vi "UART Get Bytes Available.vi"(8 "Error In":errorcluster, 10 "UART Channel (0)":u8, 11 "LINX Resource":T1) -> (0 "Error Out":errorcluster, 1 "Bytes Available":u8, 3 "LINX Resource":T1)   [LabVIEW 2020, in "LMH-LINX.lvlib"]
doc: "Get the number of bytes available in the LINX device's UART receive buffer specified by UART Channel."
uses:
  LMH-LINX.lvlib
  Private/Type Defs/LINX Ref.ctl
  Private/Type Defs/Platform.ctl
  Private/Type Defs/Interface.ctl
  Private/Device/Type Defs/LINX Device Config.ctl
  Private/Device/Type Defs/TCP Config.ctl
  Private/Device/Type Defs/Channels.ctl
  Private/Type Defs/Peripheral.ctl
  Private/Utilties/Generate Error.vi
  Private/Device/Device.lvlib
  Private/Local IO/Local IO.lvlib
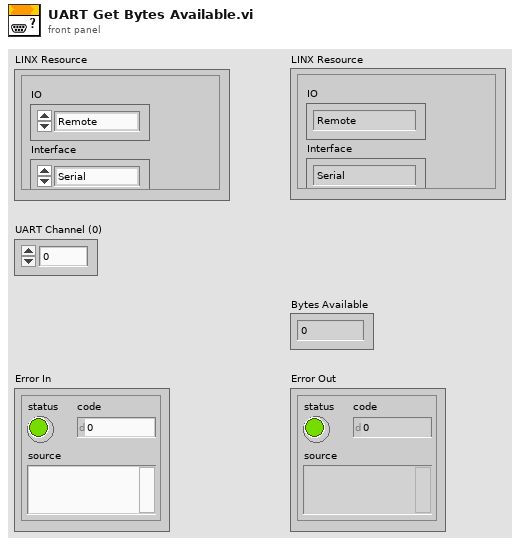
[diagram p1: front panel]
types:
  T1 = typedef "LMH-LINX.lvlib/LINX Ref.ctl" = cluster{"IO":T2, "Interface":T3, "LINX Device Config":T4}
  T2 = typedef "LMH-LINX.lvlib/Platform.ctl" = enum16{"Remote", "Local"}
  T3 = typedef "LMH-LINX.lvlib/Interface.ctl" = enum16{"Serial", "TCP"}
  T4 = typedef "Device.lvlib/LINX Device Config.ctl" = cluster{"Interface":T3, "COM Port":refnum<visa-resource-name>, "TCP Configuration":T5, "Device Family":u8, "Device ID":u8, "Device Name":string, "TCP Ref":refnum<k5>, "Channels":T6}
  T5 = typedef "Device.lvlib/TCP Config.ctl" = cluster{"IP Address":string, "Port":u16}
  T6 = typedef "LMH-LINX.lvlib/Channels.ctl" = cluster{"DI":u8[], "DO":u8[], "AI":u8[], "AO":u8[], "PWM":u8[], "QE":u8[], "UART":u8[], "I2C 2":u8[], "SPI":u8[], "CAN":u8[], "Servo":u8[], "AI Ref (V)":dbl, "AI Resolution (Bits)":u8, "AO Ref (V)":dbl, "AO Resolution (Bits)":u8}
  T7 = typedef "LMH-LINX.lvlib/Peripheral.ctl" = enum8{"DI", "DO", "AI", "AO", "PWM", "QE", "UART", "I2C", "SPI", "CAN", "Servo"}
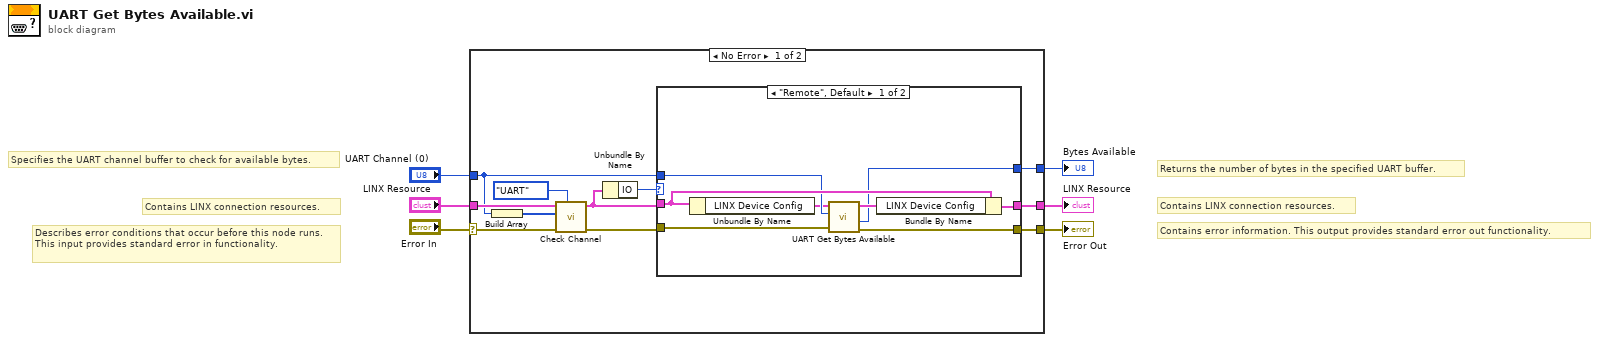
[diagram p0: block diagram]
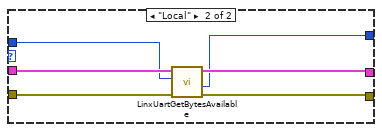
[diagram p2: hidden frame]
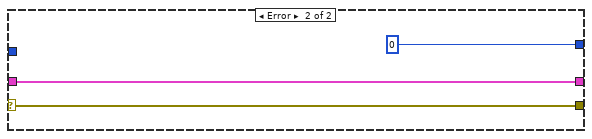
[diagram p3: hidden frame]
diagram:
  # "Returns the number of bytes in the specified UART buffer."
  # "Specifies the UART channel buffer to check for available bytes."
  # "Contains LINX connection resources."
  # "Contains error information. This output provides standard error out functionality."
  # "Contains LINX connection resources."
  # "Describes error conditions that occur before this node runs. This input provides standard error in functionality."
  n1 = case shown="No Error" "Error In" {
    selector: "Error In" -> [w7 w34]
    tunnel: [w16 w34] -> w6
    tunnel: [w15 w33] -> w5
    tunnel: "LINX Resource" -> [w14 w33]
    tunnel: "UART Channel (0)" -> [w10 _]
    tunnel: [w8 u8 0 ("Bytes at Port")] -> w2
    frame No Error {
      n2 = Build Array(w10) -> (w11:u8[])
      n3 = call "Check Channel.vi"("Peripheral"=Peripheral."UART", "Error In"=w7, "Channels"=w11, "LINX Resource"=w14) -> ("Error Out"=w12:errorcluster, "LINX Resource"=w13:T1)  [unwired: 5 in, 1 out]
      n4 = Unbundle By Name(w13) -> ("IO"=w17:T2)
      n5 = case shown="\"Remote\", Default" w17 {
        tunnel: w12 -> [w22 w31]
        tunnel: w13 -> [w25 w30]
        tunnel: [w23 w27] -> w16
        tunnel: [w24 w28] -> w15
        tunnel: w10 -> [w21 w29]
        tunnel: [w18 w26] -> w8
        frame "Remote", Default {
          n6 = Unbundle By Name(w25) -> ("LINX Device Config"=w20:T4)
          n7 = call "UART Get Bytes Available.vi"("Error In"=w22, "UART Channel"=w21, "LINX Device Config"=w20) -> ("Error Out"=w23:errorcluster, "Bytes Availabe"=w18:u8, "LINX Device Config"=w19:T4)  [unwired: 6 in]
          n8 = Bundle By Name(cluster=w25, "LINX Device Config"=w19) -> (w24:T1)
        }
        frame "Local" {
          n9 = call "LinxUartGetBytesAvailable.vi"("Error In"=w31, "Uart Channel"=w29, "LINX Resource"=w30) -> ("Error Out"=w27:errorcluster, "Num Bytes"=w26:u8, "LINX Resource"=w28:T1)  [unwired: 6 in]
        }
      }
    }
    frame Error {
    }
  }
  "Error Out" <- w6
  "LINX Resource" <- w5
  "Bytes Available" <- w2
